vi "NagleDemo-MessageSender.vi"() -> ()   [LabVIEW 2012]
panel:
  in  "TCP_NODELAY":bool=TRUE caption="false: Nagle alg. ENABLED\ntrue: Nagle alg. DISABLED"
  in  "n iterations":i32=100
  in  "IP address of MessageReflector":string
  out "value":i32
  in  "remote port":u16=5678
  out "error out":errorcluster
  out "roundtrip time (ms)":u32(graph)
  # "This VI demonstrates the effect of having the TCP Nagle algorithm enabled or disabled on  a socket for a particular kind of query/response protocol.\n\nTo run this demo, first run its partner in crime, NagleDemo-MessageSender.vi, on another machine, then run this VI after filling in the IP address of the other machine. Between runs of this VI, toggle the TCP_NODELAY boolean to see the difference."
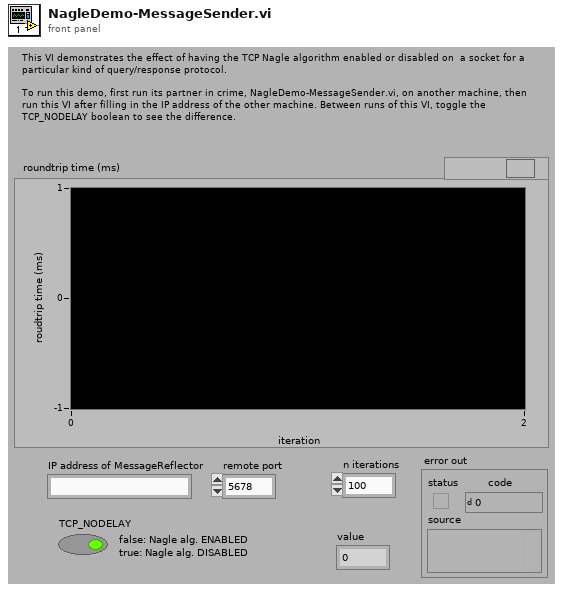
[diagram p1: front panel]
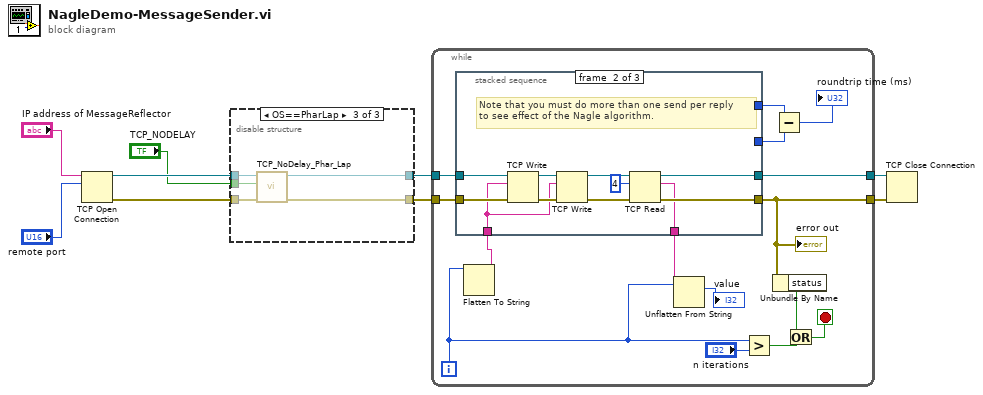
[diagram p0: block diagram]
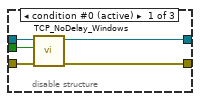
[diagram p2: hidden frame]
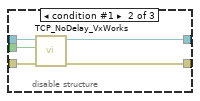
[diagram p3: hidden frame]
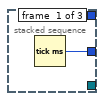
[diagram p4: hidden frame]
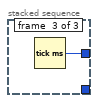
[diagram p5: hidden frame]
diagram:
  n1 = TCP Open Connection(address="IP address of MessageReflector", remote port or service name="remote port") -> (connection ID=w3:refnum<k5>, error out=w1:errorcluster)  [unwired: 3 in]
  n2 = disable-structure shown="OS==PharLap" {
    disable-tunnel: [w14 w18 w23] -> w5
    disable-tunnel: [w13 w17 w22] -> w4
    disable-tunnel: w3 -> [w12 w16 w21]
    disable-tunnel: "TCP_NODELAY" -> [w11 w15 w20]
    disable-tunnel: w1 -> [w10 w19 w24]
    frame condition #0 (active) {
      n3 = call "TCP_NoDelay_Windows.vi"("error in (no error)"=w10, "TCP_NODELAY (true)"=w11, "connID"=w12) -> ("error out"=w14:errorcluster, "connID 2"=w13:refnum<k5>)  [unwired: 3 in]
    }
    frame condition #1 {
      n4 = call "TCP_NoDelay_VxWorks.vi"("error in (no error)"=w19, "TCP_NODELAY (true)"=w15, "connID"=w16) -> ("error out"=w18:errorcluster, "connID 2"=w17:refnum<k5>)  [unwired: 3 in]
    }
    frame condition #2 {
      n5 = call "TCP_NoDelay_Phar_Lap.vi"("error in (no error)"=w24, "TCP_NODELAY (true)"=w20, "connID"=w21) -> ("error out"=w23:errorcluster, "connID 2"=w22:refnum<k5>)  [unwired: 3 in]
    }
  }
  n6 = while {
    tunnel: w4 -> [w39]
    tunnel: [w38] -> w9
    tunnel: [w34] -> w8
    tunnel: w5 -> [w37]
    i -> [w27]
    stop <- w30 stop-if-true
    n7 = Flatten To String(anything=w27) -> (data string=w29:string)  [unwired: 3 in, 2 out]
    n8 = stacked-sequence {
      tunnel: w39 -> [_ w51 _]
      tunnel: [_ w50 _] -> w38
      tunnel: w37 -> [_ w49 _]
      tunnel: [_ w47 _] -> w34
      tunnel: [w40 _ _] -> w35
      tunnel: [_ _ w52] -> w36
      tunnel: w29 -> [_ w41 _]
      tunnel: [_ w46 _] -> w28
      frame #0 {
        n9 = Tick Count (ms)() -> (millisecond timer value=w40:u32)
      }
      frame #1 {
        # "Note that you must do more than one send per reply\nto see effect of the Nagle algorithm."
        n10 = TCP Write(connection ID=w51, data in=w41, error in (no error)=w49) -> (connection ID out=w45:refnum<k5>, error out=w44:errorcluster)  [unwired: 1 in, 1 out]
        n11 = TCP Write(connection ID=w45, data in=w41, error in (no error)=w44) -> (connection ID out=w42:refnum<k5>, error out=w43:errorcluster)  [unwired: 1 in, 1 out]
        n12 = TCP Read(connection ID=w42, bytes to read=4, error in (no error)=w43) -> (connection ID out=w50:refnum<k5>, data out=w46:string, error out=w47:errorcluster)  [unwired: 2 in]
      }
      frame #2 {
        n13 = Tick Count (ms)() -> (millisecond timer value=w52:u32)
      }
    }
    "error out" <- w34
    n14 = Unflatten From String(type=w27, binary string=w28) -> (value=→"value":i32)  [unwired: 3 in, 2 out]
    n15 = Greater?(x=w27, y="n iterations") -> (0:w32:bool)
    n16 = Unbundle By Name(w34) -> ("status"=w31:bool)
    n17 = Subtract(x=w36, y=w35) -> (x-y=→"roundtrip time (ms)":u32)
    n18 = Or(x=w31, y=w32) -> (x .or. y?=w30:bool)
  }
  n19 = TCP Close Connection(connection ID=w9, error in (no error)=w8) -> ()  [unwired: 1 in, 2 out]
